vi "0-Draw Missions.vi"(8 "Image Descriptor":T1={"Upper-Left Corner Coordinates"={"UTM Zone"=0.0, "Hemisphere"=enum."North", "East"=0.0, "North"=0.0}, "Meters/Pixel"=42.294203} {"Upper-Left Corner Coordinates"."North" format="%#_10f"; "Upper-Left Corner Coordinates"."East" format="%#_8f"}, 10 "Missions":refnum<class "GenericMission.lvclass">[](array[class]), 11 "Image In":T3) -> (3 "Image Out":T3)   [LabVIEW 2011]
doc: "Overlays waypoints onto the map image."
uses:
  <vilib>/vision/Image Controls.llb/IMAQ Image.ctl
  0-Image Descriptor.ctl
  2-Think/2 Typedefs/UTM Location.ctl
  2-Think/2 Classes/Missions/GenericMission/GenericMission.lvclass
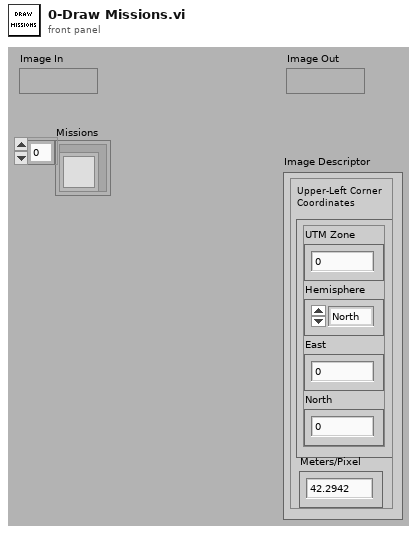
[diagram p1: front panel]
types:
  T1 = typedef "0-Image Descriptor.ctl" = cluster{"Upper-Left Corner Coordinates":T2, "Meters/Pixel":dbl}
  T2 = typedef "UTM Location.ctl" = cluster{"UTM Zone":dbl, "Hemisphere":enum16{"North", "South"}, "East":dbl, "North":dbl}
  T3 = typedef "IMAQ Image.ctl" = refnum<image>
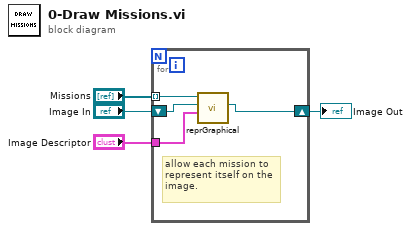
[diagram p0: block diagram]
diagram:
  n1 = for {
    shift-right: [w5] -> w3
    shift-left: "Image In" -> [w6]
    tunnel: "Image Descriptor" -> [w8]
    tunnel: "Missions" -> [w7] mode=indexing
    # "allow each mission to\nrepresent itself on the\nimage."
    n2 = call-dynamic "reprGraphical.vi"("Image Descriptor"=w8, "Image In"=w6, "GenericMission in"=w7) -> ("Image Out"=w5:T3)  [unwired: 6 in, 2 out]
  }
  "Image Out" <- w3
